vi "Generic File Dialog.vi"(6 "Selection mode":enum16{"New", "Existing", "New or Existing"}(ring), 8 "error in (no error)":errorcluster, 10 "pattern (ini files)":string="*.ini", 11 "Parameter INI File in":refnum<class "Parameter INI File.lvclass">) -> (0 "error out":errorcluster, 3 "Parameter INI File out":refnum<class "Parameter INI File.lvclass">)   [LabVIEW 2016, in "CD Parameter Manager API.lvlib" / "Parameter INI File.lvclass"]
uses:
  Parameter INI File.lvclass
  Parameter Generic File/Parameter Generic File.lvclass
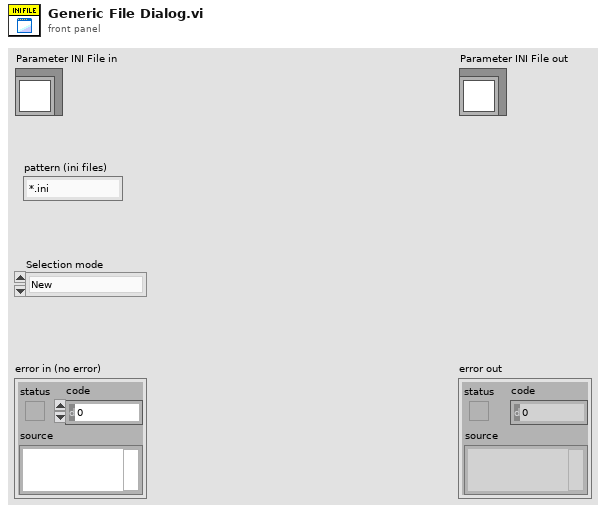
[diagram p1: front panel]
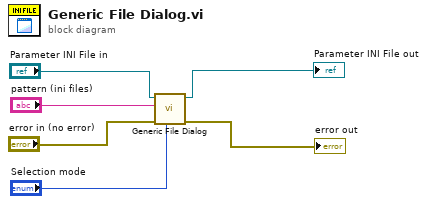
[diagram p0: block diagram]
diagram:
  n1 = call-parent "Generic File Dialog.vi"("Selection mode"="Selection mode", "error in (no error)"="error in (no error)", "pattern (all files)"="pattern (ini files)", "Parameter Generic File in"="Parameter INI File in") -> ("error out"=→"error out":errorcluster, "Parameter Generic File out"=→"Parameter INI File out":refnum<class "Parameter INI File.lvclass">)  [unwired: 6 in]
